vi "cal_sub_bool_node_pos.vi"(0 "Bool Disable Command":string="OFF", 5 "1st sub node x position":i32, 7 "Last Control  Position":cluster{"Left":i32, "Top":i32}, 9 "Last Function  Position":cluster{"Left":i32, "Top":i32}, 11 "error in":errorcluster) -> (6 "Bool Node BD Position":cluster{"1st sub node x position":i32, i32}, 15 "error out":errorcluster)   [LabVIEW 2018]
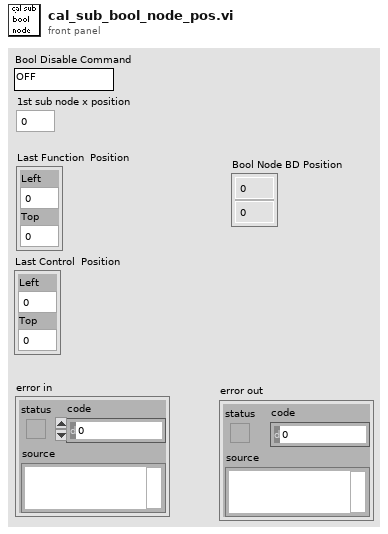
[diagram p1: front panel]
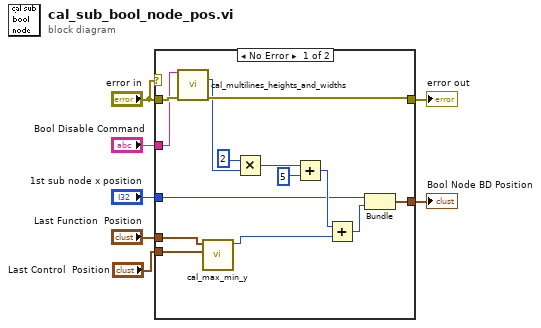
[diagram p0: block diagram]
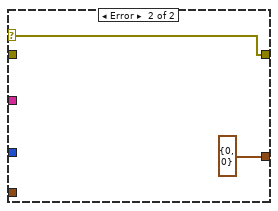
[diagram p2: hidden frame]
diagram:
  n1 = case shown="No Error" "error in" {
    selector: "error in" -> [_ w23]
    tunnel: [w21 w23] -> w7
    tunnel: "error in" -> [w20 _]
    tunnel: "Last Function  Position" -> [w10 _]
    tunnel: "Bool Disable Command" -> [w13 _]
    tunnel: "1st sub node x position" -> [w12 _]
    tunnel: [w11 cluster{"1st sub node x position":i32, i32} {"1st sub node x position"=0, 0}] -> w3
    tunnel: "Last Control  Position" -> [w9 _]
    frame No Error {
      n2 = call "cal_multilines_heights_and_widths.vi"("Ring Command"=w13, "error in (no error)"=w20) -> ("BD Height"=w15:i32, "error out"=w21:errorcluster)  [unwired: 4 in, 8 out]
      n3 = call "cal_max_min_y.vi"("Position 2"=w9, "Position 1"=w10) -> ("max y"=w8:i32)  [unwired: 9 out]
      n4 = Multiply(x=2, y=w15) -> (x*y=w17:i32)
      n5 = Add(x=w17, y=5) -> (x+y=w18:i32)
      n6 = Add(x=w18, y=w8) -> (x+y=w19:i32)
      n7 = Bundle("1st sub node x position"=w12, w19) -> (w11:cluster{"1st sub node x position":i32, i32})  [unwired: 1 out]
    }
    frame Error {
    }
  }
  "error out" <- w7
  "Bool Node BD Position" <- w3
